vi "Deadzone.vi"(1 "Deadzone":dbl, 2 "Joystick Axes In":dbl[](array[numeric])) -> (0 "Joystick Axes Out":dbl[](array[numeric]))   [LabVIEW 2014]
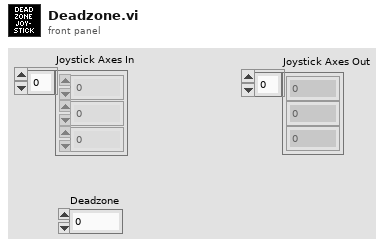
[diagram p1: front panel]
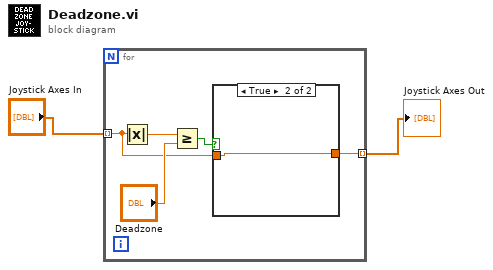
[diagram p0: block diagram]
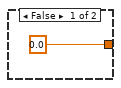
[diagram p2: hidden frame]
diagram:
  n1 = for {
    tunnel: "Joystick Axes In" -> [w3] mode=indexing
    tunnel: [w5] -> w1 mode=indexing
    n2 = Absolute Value(x=w3) -> (abs(x)=w4:dbl)
    n3 = Greater Or Equal?(x=w4, y="Deadzone") -> (x >= y?=w6:bool)
    n4 = case shown="True" w6 {
      tunnel: [0.0 w9] -> w5
      tunnel: w3 -> [_ w9]
      frame False {
      }
      frame True {
      }
    }
  }
  "Joystick Axes Out" <- w1
